vi "POP_Create Search Names.vi"(9 "Column String":string="1", 10 "Tag or Row String":string="12123", 11 "Control Ref String":string="-277872553") -> (3 "Search Names":string[](array[string])=["-277872553/12123/1\r\n", "-277872553//1\r\n", "-277872553/12123/\r\n", "-277872553//\r\n"])   [LabVIEW 2016]
panel:
  out "Ctl Code":string="-277872553//\r\n"
  out "Row Code":string="-277872553/12123/\r\n"
  out "Column Code":string="-277872553//1\r\n"
  out "Cell Code":string="-277872553/12123/1\r\n"
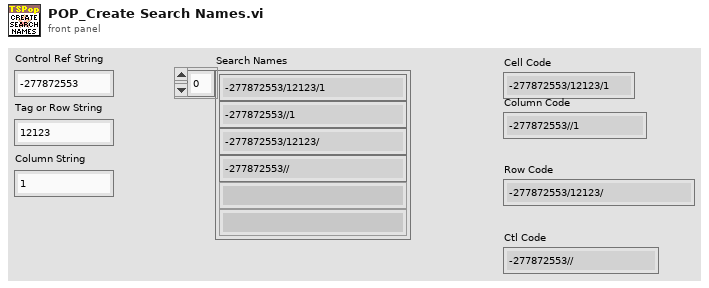
[diagram p1: front panel]
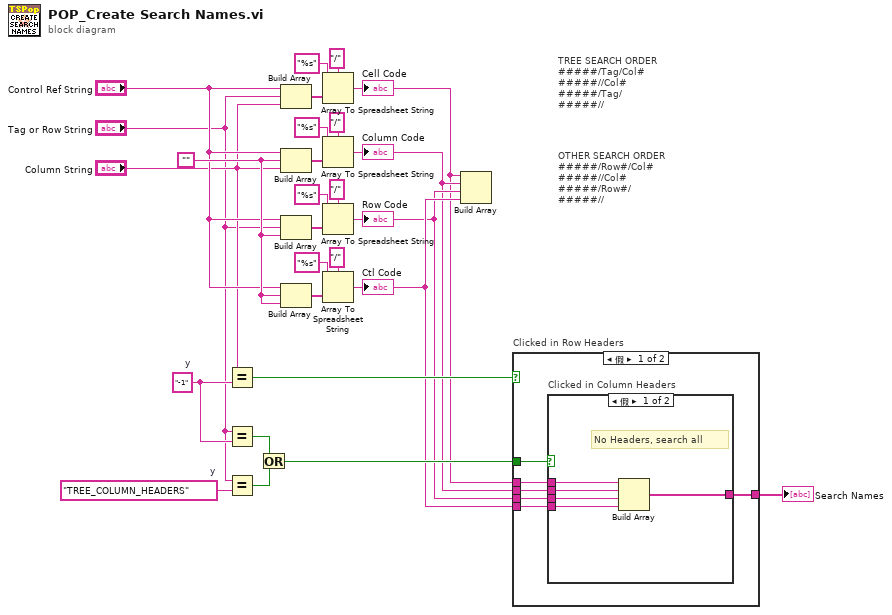
[diagram p0: block diagram]
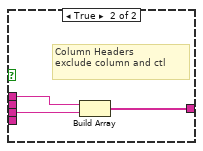
[diagram p2: hidden frame]
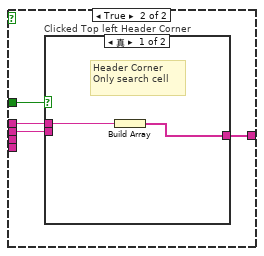
[diagram p3: hidden frame]
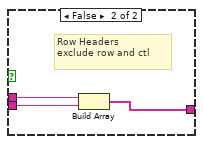
[diagram p4: hidden frame]
diagram:
  w11 = "-1"  # y
  w9 = "TREE_COLUMN_HEADERS"  # y
  w15 = ""
  # "OTHER SEARCH ORDER\n#####/Row#/Col#\n#####//Col#\n#####/Row#/\n#####//"
  # "TREE SEARCH ORDER\n#####/Tag/Col#\n#####//Col#\n#####/Tag/\n#####//"
  n1 = Equal?(x="Column String", y=w11) -> (x = y?=w13:bool)
  n2 = Equal?(x="Tag or Row String", y=w11) -> (x = y?=w8:bool)
  n3 = Equal?(x="Tag or Row String", y=w9) -> (x = y?=w7:bool)
  n4 = Or(x=w8, y=w7) -> (x .or. y?=w6:bool)
  n5 = Build Array("Control Ref String", "Tag or Row String", "Column String") -> (w27:string[])
  n6 = Build Array("Control Ref String", w15, "Column String") -> (w22:string[])
  n7 = Build Array("Control Ref String", "Tag or Row String", w15) -> (w21:string[])
  n8 = Build Array("Control Ref String", w15, w15) -> (w16:string[])
  n9 = Array To Spreadsheet String(delimiter (Tab)="/", array=w27, 3:"%s" ("format string")) -> (spreadsheet string=w2:string)
  "Cell Code" <- w2
  n10 = Array To Spreadsheet String(delimiter (Tab)="/", array=w22, 3:"%s" ("format string")) -> (spreadsheet string=w3:string)
  "Column Code" <- w3
  n11 = Array To Spreadsheet String(delimiter (Tab)="/", array=w21, 3:"%s" ("format string")) -> (spreadsheet string=w4:string)
  "Row Code" <- w4
  n12 = Array To Spreadsheet String(delimiter (Tab)="/", array=w16, 3:"%s" ("format string")) -> (spreadsheet string=w5:string)
  "Ctl Code" <- w5
  n13 = Build Array(w2, w3, w4, w5) -> ()  [unwired: 1 out]
  n14 = case "Clicked in Row Headers" shown="假" w13 {
    tunnel: w6 -> [w33 w45]
    tunnel: w5 -> [w32 _]
    tunnel: w4 -> [w31 _]
    tunnel: w3 -> [w30 w42]
    tunnel: w2 -> [w29 w44]
    tunnel: [w28 w43] -> w1
    frame False {
      n15 = case "Clicked in Column Headers" shown="假" w33 {
        tunnel: w32 -> [w38 _]
        tunnel: w31 -> [w37 w41]
        tunnel: w30 -> [w36 _]
        tunnel: w29 -> [w35 w40]
        tunnel: [w34 w39] -> w28
        frame False {
          # "No Headers, search all"
          n16 = Build Array(w35, w36, w37, w38) -> (w34:string[])
        }
        frame True {
          # "Column Headers\nexclude column and ctl"
          n17 = Build Array(w40, w41) -> (w39:string[])
        }
      }
    }
    frame True {
      n18 = case "Clicked Top left Header Corner" shown="真" w45 {
        tunnel: w44 -> [w47 w50]
        tunnel: [w46 w49] -> w43
        tunnel: w42 -> [_ w48]
        frame True {
          # "Header Corner\nOnly search cell"
          n19 = Build Array(w47) -> (w46:string[])
        }
        frame False {
          # "Row Headers\nexclude row and ctl"
          n20 = Build Array(w50, w48) -> (w49:string[])
        }
      }
    }
  }
  "Search Names" <- w1
